vi "Create DAQ Task.vi"(8 "error in":errorcluster, 9 "User provided rate":dbl, 10 "Search for Max rate? (F)":bool, 11 "Channels":T1[](array[typedef]) format="%.0x") -> (0 "error out":errorcluster, 1 "Actual rate":dbl, 3 "task out":refnum<k21>)   [LabVIEW 2011, in "PXIe-433x Custom Device.lvlib"]
uses:
  PXIe-433x Custom Device.lvlib
  <vilib>/NI Veristand/Custom Device API/Custom Device Item Ref.ctl
  Sensor Type.ctl
  Strain Information.ctl
  Strain Bridge Information.ctl
  Scale Type.ctl
  Global.vi
  <vilib>/NI Veristand/Custom Device API/Get Item Property (Variant).vi
  <vilib>/NI Veristand/Custom Device API/Get Item Property (Double).vi
  <vilib>/NI Veristand/Custom Device API/Get Item Property (U16).vi
  <vilib>/DAQmx/create/channels.llb/DAQmx Create Channel (AI-Strain-Strain Gage).vi
  <vilib>/DAQmx/create/channels.llb/DAQmx Create Channel (AI-Force-Bridge-Two-Point-Linear).vi
  <vilib>/DAQmx/create/channels.llb/DAQmx Create Channel (AI-Force-Bridge-Table).vi
  <vilib>/DAQmx/create/channels.llb/DAQmx Create Channel (AI-Force-Bridge-Polynomial).vi
  <vilib>/DAQmx/create/channels.llb/DAQmx Create Channel (AI-Pressure-Bridge-Two-Point-Linear).vi
  <vilib>/DAQmx/create/channels.llb/DAQmx Create Channel (AI-Pressure-Bridge-Table).vi
  <vilib>/DAQmx/create/channels.llb/DAQmx Create Channel (AI-Pressure-Bridge-Polynomial).vi
  <vilib>/DAQmx/create/channels.llb/DAQmx Create Channel (AI-Torque-Bridge-Two-Point-Linear).vi
  <vilib>/DAQmx/create/channels.llb/DAQmx Create Channel (AI-Torque-Bridge-Table).vi
  <vilib>/DAQmx/create/channels.llb/DAQmx Create Channel (AI-Torque-Bridge-Polynomial).vi
  <vilib>/NI Veristand/Custom Device API/Custom Device API.lvlib
  Program Files (x86)/National Instruments/LabVIEW 2011/resource/objmgr/daqmx.rc
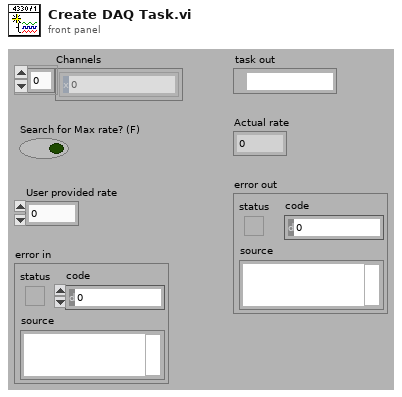
[diagram p1: front panel]
types:
  T1 = typedef "Custom Device API.lvlib/Custom Device Item Ref.ctl" = u64
  T2 = typedef "PXIe-433x Custom Device.lvlib/Sensor Type.ctl" = enum16{"Strain", "Force", "Pressure", "Torque"}
  T3 = typedef "PXIe-433x Custom Device.lvlib/Strain Bridge Information.ctl" = cluster{"strain configuration":i32, "lead wire resistance":dbl, "initial bridge voltage":dbl, "voltage excitation source":i32, "voltage excitation value":dbl}
  T4 = cluster{"bridge configuration":i32, "voltage excitation source":i32, "voltage excitation value":dbl, "nominal bridge resistance":dbl}
  T5 = cluster{"first electrical value":dbl, "second electrical value":dbl, "electrical units":i32, "first physical value":dbl, "second physical value":dbl, "physical units":i32}
  T6 = cluster{"electrical values":dbl[], "electrical units":i32, "physical values":dbl[], "physical units":i32}
  T7 = cluster{"forward coeff":dbl[], "reverse coeff":dbl[], "electrical units":i32, "physical units":i32}
  T8 = typedef "Custom Device API.lvlib/Custom Device Item Info.ctl" = cluster{"Name":string, "Is Channel":bool, "GUID":string}
  T9 = typedef "PXIe-433x Custom Device.lvlib/Strain Information.ctl" = cluster{"gage factor":dbl, "nominal gage resistance":dbl, "poisson ratio":dbl}
  T10 = typedef "PXIe-433x Custom Device.lvlib/Scale Type.ctl" = enum16{"Linear", "Table", "Polynomial"}
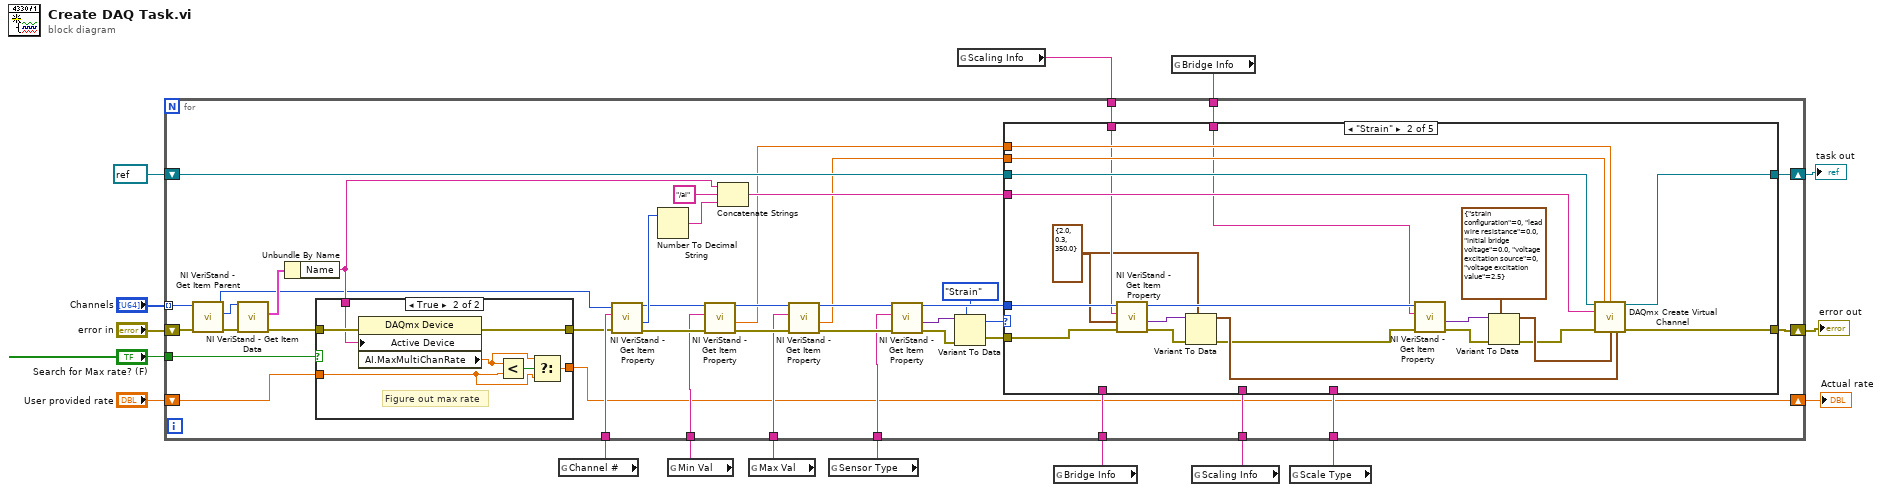
[diagram p0: block diagram]
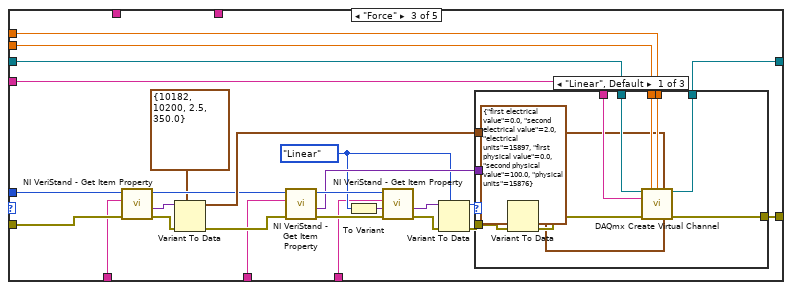
[diagram p4: hidden frame]
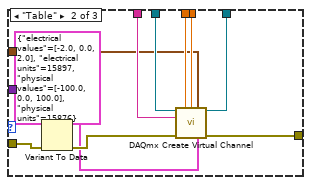
[diagram p5: hidden frame]
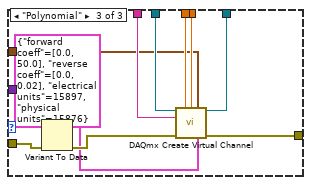
[diagram p6: hidden frame]
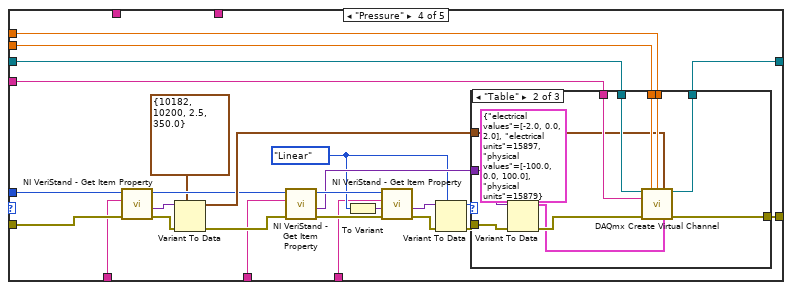
[diagram p7: hidden frame]
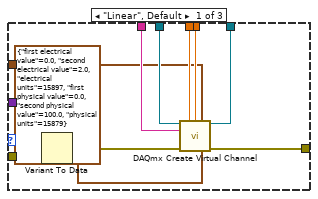
[diagram p8: hidden frame]
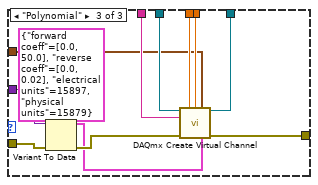
[diagram p9: hidden frame]
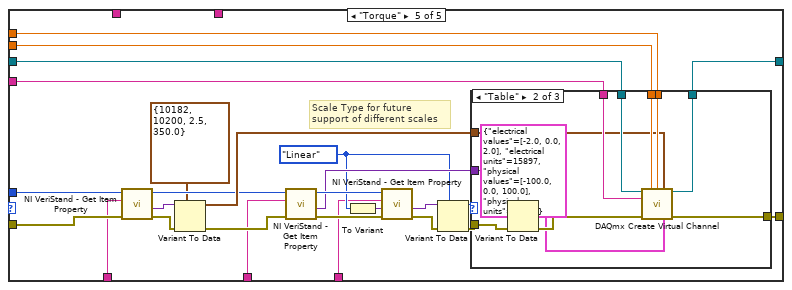
[diagram p10: hidden frame]
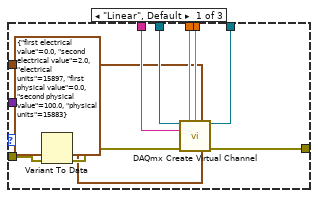
[diagram p11: hidden frame]
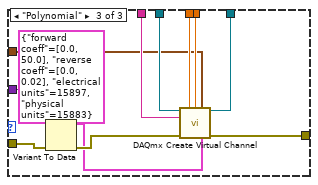
[diagram p12: hidden frame]
diagram:
  n1 = global read "Global.vi" "Channel #"() -> (w6:string)
  n2 = global read "Global.vi" "Min Val"() -> (w7:string)
  n3 = global read "Global.vi" "Max Val"() -> (w8:string)
  n4 = global read "Global.vi" "Sensor Type"() -> (w9:string)
  n5 = global read "Global.vi" "Scaling Info"() -> (w10:string)
  n6 = global read "Global.vi" "Bridge Info"() -> (w12:string)
  n7 = global read "Global.vi" "Bridge Info"() -> (w11:string)
  n8 = global read "Global.vi" "Scaling Info"() -> (w13:string)
  n9 = global read "Global.vi" "Scale Type"() -> (w14:string)
  n10 = for {
    tunnel: "Channels" -> [w37] mode=indexing
    shift-right: [w53] -> w1
    shift-left: "error in" -> [w38]
    shift-right: [w59] -> w2
    shift-left: refnum<k21> refnum ("task out") -> [w58]
    tunnel: w6 -> [w33]
    tunnel: w7 -> [w32]
    tunnel: w8 -> [w31]
    tunnel: w9 -> [w30]
    tunnel: w10 -> [w26]
    tunnel: w11 -> [w25]
    tunnel: w12 -> [w24]
    tunnel: w13 -> [w23]
    tunnel: w14 -> [w22]
    shift-right: [w20] -> w15
    shift-left: "User provided rate" -> [w21]
    tunnel: "Search for Max rate? (F)" -> [w18]
    n11 = call <vilib>:"NI VeriStand - Get Item Parent.vi"("error in (no error)"=w38, "Item Ref in"=w37) -> ("error out"=w36:errorcluster, "Parent Ref"=w35:T1, "Item Ref out"=w19:T1)  [unwired: 6 in, 1 out]
    n12 = call <vilib>:"NI VeriStand - Get Item Data.vi"("error in (no error)"=w36, "Item Ref in"=w35) -> ("error out"=w29:errorcluster, "Item Info"=w34:T8)  [unwired: 6 in, 2 out]
    n13 = Unbundle By Name(w34) -> ("Name"=w28:string)
    n14 = case shown="True" w18 {
      tunnel: w29 -> [w61 w68]
      tunnel: w28 -> [_ w67]
      tunnel: [w61 w66] -> w27
      tunnel: w21 -> [w60 w65]
      tunnel: [w60 w64] -> w20
      frame False {
        # "Use whatever they set"
      }
      frame True {
        # "Figure out max rate"
        n15 = property class="DAQmx Device"(error in=w68, "Active Device"=w67) -> (error out=w66:errorcluster, "AI.MaxMultiChanRate"=w62:dbl)  [unwired: 1 in, 1 out]
        n16 = Less?(x=w62, y=w65) -> (x < y?=w63:bool)
        n17 = Select(t=w62, s=w63, f=w65) -> (s? t:f=w64:dbl)
      }
    }
    n18 = call-poly <vilib>:"NI VeriStand - Get Item Property.vi"("error in (no error)"=w27, "Property Name"=w33, "Item Ref in"=w19) -> ("error out"=w44:errorcluster, "Value"=w57:u16, "Item Ref out"=w43:T1)  [unwired: 5 in, 1 out]
    n19 = Number To Decimal String(number=w57) -> (decimal integer string=w55:string)  [unwired: 1 in]
    n20 = call-poly <vilib>:"NI VeriStand - Get Item Property.vi"("error in (no error)"=w44, "Property Name"=w32, "Item Ref in"=w43) -> ("error out"=w46:errorcluster, "Value"=w40:dbl, "Item Ref out"=w45:T1)  [unwired: 5 in, 1 out]
    n21 = Concatenate Strings(w28, "/ai" ("string"), w55) -> (w56:string)
    n22 = call-poly <vilib>:"NI VeriStand - Get Item Property.vi"("error in (no error)"=w46, "Property Name"=w31, "Item Ref in"=w45) -> ("error out"=w41:errorcluster, "Value"=w39:dbl, "Item Ref out"=w42:T1)  [unwired: 5 in, 1 out]
    n23 = call-poly <vilib>:"NI VeriStand - Get Item Property.vi"("error in (no error)"=w41, "Property Name"=w30, "Item Ref in"=w42) -> ("error out"=w51:errorcluster, "Value"=w47:variant, "Item Ref out"=w52:T1)  [unwired: 5 in, 1 out]
    n24 = Variant To Data(error in=w51, type=Sensor_Type."Strain" ("Sensor Type"), Variant=w47) -> (data=w48:T2, error out=w50:errorcluster)
    n25 = case shown="\"Strain\"" w48 {
      tunnel: [w69 w91 w117 w179 w241] -> w59
      tunnel: w58 -> [w69 w90 w116 w178 w240]
      tunnel: w56 -> [_ w89 w115 w177 w239]
      tunnel: [w70 w87 w114 w176 w238] -> w53
      tunnel: w52 -> [_ w78 w109 w171 w233]
      tunnel: w50 -> [w70 w77 w108 w170 w232]
      tunnel: w40 -> [_ w75 w106 w168 w230]
      tunnel: w39 -> [_ w74 w105 w167 w229]
      tunnel: w26 -> [_ w73 _ _ _]
      tunnel: w25 -> [_ w72 _ _ _]
      tunnel: w24 -> [_ _ w94 w156 w218]
      tunnel: w23 -> [_ _ w93 w155 w217]
      tunnel: w22 -> [_ _ w92 w154 w216]
      frame Default {
      }
      frame "Strain" {
        w71 = T9 {"gage factor"=2.0, "nominal gage resistance"=0.3, "poisson ratio"=350.0} ("strain gage information")
        n26 = call-poly <vilib>:"NI VeriStand - Get Item Property.vi"("error in (no error)"=w77, "Default Value"=w71, "Property Name"=w73, "Item Ref in"=w78) -> ("error out"=w81:errorcluster, "Value"=w83:variant, "Item Ref out"=w88:T1)  [unwired: 4 in, 1 out]
        n27 = Variant To Data(error in=w81, type=w71, Variant=w83) -> (data=w82:T9, error out=w80:errorcluster)
        n28 = call-poly <vilib>:"NI VeriStand - Get Item Property.vi"("error in (no error)"=w80, "Property Name"=w72, "Item Ref in"=w88) -> ("error out"=w79:errorcluster, "Value"=w86:variant)  [unwired: 5 in, 2 out]
        n29 = Variant To Data(error in=w79, type=T3 {"strain configuration"=0, "lead wire resistance"=0.0, "initial bridge voltage"=0.0, "voltage excitation source"=0, "voltage excitation value"=2.5} ("bridge information"), Variant=w86) -> (data=w84:T3, error out=w76:errorcluster)
        n30 = call-poly <vilib>:"DAQmx Create Virtual Channel.vi"("task in"=w90, "maximum value"=w74, "minimum value"=w75, "physical channels"=w89, "error in"=w76, "bridge information"=w84, "strain gage information"=w82) -> ("task out"=w91:refnum<k21>, "error out"=w87:errorcluster)  [unwired: 7 in]
      }
      frame "Force" {
        w96 = Scale_Type."Linear" ("Scale Type")
        n31 = call-poly <vilib>:"NI VeriStand - Get Item Property.vi"("error in (no error)"=w108, "Property Name"=w94, "Item Ref in"=w109) -> ("error out"=w111:errorcluster, "Value"=w112:variant, "Item Ref out"=w102:T1)  [unwired: 5 in, 1 out]
        n32 = Variant To Data(error in=w111, type=T4 {"bridge configuration"=10182, "voltage excitation source"=10200, "voltage excitation value"=2.5, "nominal bridge resistance"=350.0} ("bridge information"), Variant=w112) -> (data=w104:T4, error out=w99:errorcluster)
        n33 = call-poly <vilib>:"NI VeriStand - Get Item Property.vi"("error in (no error)"=w99, "Property Name"=w93, "Item Ref in"=w102) -> ("error out"=w100:errorcluster, "Value"=w98:variant, "Item Ref out"=w101:T1)  [unwired: 5 in, 1 out]
        n34 = To Variant(anything=w96) -> (Variant=w97:variant)
        n35 = call-poly <vilib>:"NI VeriStand - Get Item Property.vi"("error in (no error)"=w100, "Default Value"=w97, "Property Name"=w92, "Item Ref in"=w101) -> ("error out"=w110:errorcluster, "Value"=w113:variant)  [unwired: 4 in, 2 out]
        n36 = Variant To Data(error in=w110, type=w96, Variant=w113) -> (data=w103:T10, error out=w107:errorcluster)
        n37 = case shown="\"Linear\", Default" w103 {
          tunnel: [w129 w141 w153] -> w117
          tunnel: w116 -> [w128 w140 w152]
          tunnel: w115 -> [w127 w139 w151]
          tunnel: [w126 w138 w150] -> w114
          tunnel: w107 -> [w122 w134 w146]
          tunnel: w106 -> [w125 w137 w149]
          tunnel: w105 -> [w124 w136 w148]
          tunnel: w104 -> [w123 w135 w147]
          tunnel: w98 -> [w120 w132 w144]
          frame "Linear", Default {
            n38 = Variant To Data(error in=w122, type=T5 {"first electrical value"=0.0, "second electrical value"=2.0, "electrical units"=15897, "first physical value"=0.0, "second physical value"=100.0, "physical units"=15876} ("scaling information"), Variant=w120) -> (data=w118:T5, error out=w121:errorcluster)
            n39 = call-poly <vilib>:"DAQmx Create Virtual Channel.vi"("task in"=w128, "maximum value"=w124, "minimum value"=w125, "bridge information"=w123, "physical channels"=w127, "error in"=w121, "scaling information"=w118) -> ("task out"=w129:refnum<k21>, "error out"=w126:errorcluster)  [unwired: 7 in]
          }
          frame "Table" {
            n40 = Variant To Data(error in=w134, type=T6 {"electrical values"=[-2.0, 0.0, 2.0], "electrical units"=15897, "physical values"=[-100.0, 0.0, 100.0], "physical units"=15876} ("scaling information"), Variant=w132) -> (data=w131:T6, error out=w133:errorcluster)
            n41 = call-poly <vilib>:"DAQmx Create Virtual Channel.vi"("task in"=w140, "maximum value"=w136, "minimum value"=w137, "bridge information"=w135, "physical channels"=w139, "error in"=w133, "scaling information"=w131) -> ("task out"=w141:refnum<k21>, "error out"=w138:errorcluster)  [unwired: 7 in]
          }
          frame "Polynomial" {
            n42 = Variant To Data(error in=w146, type=T7 {"forward coeff"=[0.0, 50.0], "reverse coeff"=[0.0, 0.02], "electrical units"=15897, "physical units"=15876} ("scaling information"), Variant=w144) -> (data=w143:T7, error out=w145:errorcluster)
            n43 = call-poly <vilib>:"DAQmx Create Virtual Channel.vi"("task in"=w152, "maximum value"=w148, "minimum value"=w149, "bridge information"=w147, "physical channels"=w151, "error in"=w145, "scaling information"=w143) -> ("task out"=w153:refnum<k21>, "error out"=w150:errorcluster)  [unwired: 7 in]
          }
        }
      }
      frame "Pressure" {
        w158 = Scale_Type."Linear" ("Scale Type")
        n44 = call-poly <vilib>:"NI VeriStand - Get Item Property.vi"("error in (no error)"=w170, "Property Name"=w156, "Item Ref in"=w171) -> ("error out"=w173:errorcluster, "Value"=w174:variant, "Item Ref out"=w164:T1)  [unwired: 5 in, 1 out]
        n45 = Variant To Data(error in=w173, type=T4 {"bridge configuration"=10182, "voltage excitation source"=10200, "voltage excitation value"=2.5, "nominal bridge resistance"=350.0} ("bridge information"), Variant=w174) -> (data=w166:T4, error out=w161:errorcluster)
        n46 = call-poly <vilib>:"NI VeriStand - Get Item Property.vi"("error in (no error)"=w161, "Property Name"=w155, "Item Ref in"=w164) -> ("error out"=w162:errorcluster, "Value"=w160:variant, "Item Ref out"=w163:T1)  [unwired: 5 in, 1 out]
        n47 = To Variant(anything=w158) -> (Variant=w159:variant)
        n48 = call-poly <vilib>:"NI VeriStand - Get Item Property.vi"("error in (no error)"=w162, "Default Value"=w159, "Property Name"=w154, "Item Ref in"=w163) -> ("error out"=w172:errorcluster, "Value"=w175:variant)  [unwired: 4 in, 2 out]
        n49 = Variant To Data(error in=w172, type=w158, Variant=w175) -> (data=w165:T10, error out=w169:errorcluster)
        n50 = case shown="\"Table\"" w165 {
          tunnel: [w191 w203 w215] -> w179
          tunnel: w178 -> [w190 w202 w214]
          tunnel: w177 -> [w189 w201 w213]
          tunnel: [w188 w200 w212] -> w176
          tunnel: w169 -> [w184 w196 w208]
          tunnel: w168 -> [w187 w199 w211]
          tunnel: w167 -> [w186 w198 w210]
          tunnel: w166 -> [w185 w197 w209]
          tunnel: w160 -> [w182 w194 w206]
          frame "Linear", Default {
            n51 = Variant To Data(error in=w184, type=T5 {"first electrical value"=0.0, "second electrical value"=2.0, "electrical units"=15897, "first physical value"=0.0, "second physical value"=100.0, "physical units"=15879} ("scaling information"), Variant=w182) -> (data=w181:T5, error out=w183:errorcluster)
            n52 = call-poly <vilib>:"DAQmx Create Virtual Channel.vi"("task in"=w190, "maximum value"=w186, "minimum value"=w187, "bridge information"=w185, "physical channels"=w189, "error in"=w183, "scaling information"=w181) -> ("task out"=w191:refnum<k21>, "error out"=w188:errorcluster)  [unwired: 7 in]
          }
          frame "Table" {
            n53 = Variant To Data(error in=w196, type=T6 {"electrical values"=[-2.0, 0.0, 2.0], "electrical units"=15897, "physical values"=[-100.0, 0.0, 100.0], "physical units"=15879} ("scaling information"), Variant=w194) -> (data=w193:T6, error out=w195:errorcluster)
            n54 = call-poly <vilib>:"DAQmx Create Virtual Channel.vi"("task in"=w202, "maximum value"=w198, "minimum value"=w199, "bridge information"=w197, "physical channels"=w201, "error in"=w195, "scaling information"=w193) -> ("task out"=w203:refnum<k21>, "error out"=w200:errorcluster)  [unwired: 7 in]
          }
          frame "Polynomial" {
            n55 = Variant To Data(error in=w208, type=T7 {"forward coeff"=[0.0, 50.0], "reverse coeff"=[0.0, 0.02], "electrical units"=15897, "physical units"=15879} ("scaling information"), Variant=w206) -> (data=w205:T7, error out=w207:errorcluster)
            n56 = call-poly <vilib>:"DAQmx Create Virtual Channel.vi"("task in"=w214, "maximum value"=w210, "minimum value"=w211, "bridge information"=w209, "physical channels"=w213, "error in"=w207, "scaling information"=w205) -> ("task out"=w215:refnum<k21>, "error out"=w212:errorcluster)  [unwired: 7 in]
          }
        }
      }
      frame "Torque" {
        w220 = Scale_Type."Linear" ("Scale Type")
        # "Scale Type for future support of different scales"
        n57 = call-poly <vilib>:"NI VeriStand - Get Item Property.vi"("error in (no error)"=w232, "Property Name"=w218, "Item Ref in"=w233) -> ("error out"=w235:errorcluster, "Value"=w236:variant, "Item Ref out"=w226:T1)  [unwired: 5 in, 1 out]
        n58 = Variant To Data(error in=w235, type=T4 {"bridge configuration"=10182, "voltage excitation source"=10200, "voltage excitation value"=2.5, "nominal bridge resistance"=350.0} ("bridge information"), Variant=w236) -> (data=w228:T4, error out=w223:errorcluster)
        n59 = call-poly <vilib>:"NI VeriStand - Get Item Property.vi"("error in (no error)"=w223, "Property Name"=w217, "Item Ref in"=w226) -> ("error out"=w224:errorcluster, "Value"=w222:variant, "Item Ref out"=w225:T1)  [unwired: 5 in, 1 out]
        n60 = To Variant(anything=w220) -> (Variant=w221:variant)
        n61 = call-poly <vilib>:"NI VeriStand - Get Item Property.vi"("error in (no error)"=w224, "Default Value"=w221, "Property Name"=w216, "Item Ref in"=w225) -> ("error out"=w234:errorcluster, "Value"=w237:variant)  [unwired: 4 in, 2 out]
        n62 = Variant To Data(error in=w234, type=w220, Variant=w237) -> (data=w227:T10, error out=w231:errorcluster)
        n63 = case shown="\"Table\"" w227 {
          tunnel: [w253 w265 w277] -> w241
          tunnel: w240 -> [w252 w264 w276]
          tunnel: w239 -> [w251 w263 w275]
          tunnel: [w250 w262 w274] -> w238
          tunnel: w231 -> [w246 w259 w270]
          tunnel: w230 -> [w249 w261 w273]
          tunnel: w229 -> [w248 w260 w272]
          tunnel: w228 -> [w247 w254 w271]
          tunnel: w222 -> [w244 w257 w268]
          frame "Linear", Default {
            n64 = Variant To Data(error in=w246, type=T5 {"first electrical value"=0.0, "second electrical value"=2.0, "electrical units"=15897, "first physical value"=0.0, "second physical value"=100.0, "physical units"=15883} ("scaling information"), Variant=w244) -> (data=w243:T5, error out=w245:errorcluster)
            n65 = call-poly <vilib>:"DAQmx Create Virtual Channel.vi"("task in"=w252, "maximum value"=w248, "minimum value"=w249, "bridge information"=w247, "physical channels"=w251, "error in"=w245, "scaling information"=w243) -> ("task out"=w253:refnum<k21>, "error out"=w250:errorcluster)  [unwired: 7 in]
          }
          frame "Table" {
            n66 = Variant To Data(error in=w259, type=T6 {"electrical values"=[-2.0, 0.0, 2.0], "electrical units"=15897, "physical values"=[-100.0, 0.0, 100.0], "physical units"=15883} ("scaling information"), Variant=w257) -> (data=w256:T6, error out=w258:errorcluster)
            n67 = call-poly <vilib>:"DAQmx Create Virtual Channel.vi"("task in"=w264, "maximum value"=w260, "minimum value"=w261, "bridge information"=w254, "physical channels"=w263, "error in"=w258, "scaling information"=w256) -> ("task out"=w265:refnum<k21>, "error out"=w262:errorcluster)  [unwired: 7 in]
          }
          frame "Polynomial" {
            n68 = Variant To Data(error in=w270, type=T7 {"forward coeff"=[0.0, 50.0], "reverse coeff"=[0.0, 0.02], "electrical units"=15897, "physical units"=15883} ("scaling information"), Variant=w268) -> (data=w267:T7, error out=w269:errorcluster)
            n69 = call-poly <vilib>:"DAQmx Create Virtual Channel.vi"("task in"=w276, "maximum value"=w272, "minimum value"=w273, "bridge information"=w271, "physical channels"=w275, "error in"=w269, "scaling information"=w267) -> ("task out"=w277:refnum<k21>, "error out"=w274:errorcluster)  [unwired: 7 in]
          }
        }
      }
    }
  }
  "Actual rate" <- w15
  "task out" <- w2
  "error out" <- w1
